vi "Main.vi"() -> ()   [LabVIEW 2017]
uses:
  Controls/Timing Controls.ctl
  Controls/File Controls.ctl
  Controls/DAQ State.ctl
  <vilib>/DAQmx/write.llb/DAQmx Write (Analog 1D DBL NChan 1Samp).vi
  <vilib>/DAQmx/configure/timing.llb/DAQmx Timing (Sample Clock).vi
  <vilib>/DAQmx/miscellaneous.llb/DAQmx Fill In Error Info.vi
panel:
  in  "Single Channel?":bool
  in  "Lower Limit":dbl=-0.85
  in  "Upper Limit":dbl=-0.75
  out "Differential":cluster{dbl[], dbl[]}[](graph)=[{[0.0, 1.0], [0.0029010882279960626, 0.00862868344710327]}, {[-1.0, 2.0], [-0.75, -0.75]}, {[-1.0, 2.0], [-0.85, -0.85]}]
  out "Saving?":bool
  out "Zero Values Dev2":dbl[](array[numeric])
  out "Zero Values Dev1":dbl[](array[numeric])
  in  "Save":bool
  in  "File Control":T1={"File Path"=path "C:/Users/localadmin/Documents/Acquisition Data", "File Name"=""}
  out "Trigger":dynamicdata(graph)=[{"t0"=timestamp(3616576961.7901273 s since 1904-01-01), "dt"=0.001, "Y"=[2.8935987566836108, 2.892940411376444, 2.8932695840305964, 2.8932695840305964, 2.8932695840305964, 2.8932695840305964, 2.8934341703572457, 2.8935987566836108, 2.8935987566836108, 2.893763343009691, 2.8934341703572457, 2.8940925156609985, 2.8940925156609985, 2.8942571019862253, 2.8940925156609985, 2.8935987566836108, 2.893927929335487, 2.893763343009691, 2.893763343009691, 2.8934341703572457, 2.8932695840305964, 2.8932695840305964, 2.8931049977036625, 2.8934341703572457, 2.8931049977036625, 2.8932695840305964, 2.8931049977036625, 2.8935987566836108, 2.893927929335487, 2.893927929335487, 2.893763343009691, 2.8942571019862253, 2.8942571019862253, 2.8940925156609985, 2.893927929335487, 2.893927929335487, 2.893763343009691, 2.893763343009691, 2.8935987566836108, 2.8932695840305964, 2.8934341703572457, 2.892775825048941, 2.8931049977036625, 2.892940411376444, 2.8931049977036625, 2.8934341703572457, 2.8934341703572457, 2.893763343009691, 2.893763343009691, 2.893927929335487, 2.893763343009691, 2.894421688311168, 2.8942571019862253, 2.894421688311168, 2.8940925156609985, 2.893927929335487, 2.894421688311168, 2.894421688311168, 2.893763343009691, 2.8934341703572457, 2.893927929335487, 2.892940411376444, 2.8935987566836108, 2.8931049977036625, 2.8934341703572457, 2.8935987566836108, 2.8935987566836108, 2.893763343009691, 2.893763343009691, 2.8942571019862253, 2.893927929335487, 2.894421688311168, 2.8947508609601993, 2.894421688311168, 2.8940925156609985, 2.8940925156609985, 2.8942571019862253, 2.8940925156609985, 2.893763343009691, 2.8935987566836108, 2.8934341703572457, 2.8931049977036625, 2.892940411376444, 2.8931049977036625, 2.8932695840305964, 2.8931049977036625, 2.8932695840305964, 2.8935987566836108, 2.8935987566836108, 2.8942571019862253, 2.893927929335487, 2.894421688311168, 2.893927929335487, 2.894586274635826, 2.893927929335487, 2.8942571019862253, 2.893927929335487, 2.8940925156609985, 2.893763343009691, 2.8932695840305964], "attributes"=variant("NI_ChannelName"=variant(string "Trigger"), "NI_UnitDescription"=variant(string "Volts"))}]
  out "Dev1":dynamicdata(graph)=[{"t0"=timestamp(3616576961.790079 s since 1904-01-01), "dt"=0.001, "Y"=[0.004713341620051992, 0.0045485913126213084, 0.005042842234350253, 0.0052075925412182755, 0.004219090697197281, 0.0038895900810222983, 0.004219090697197281, 0.0043838410050032195, 0.0038895900810222983, 0.0037248397726536986, 0.004713341620051992, 0.0045485913126213084, 0.0045485913126213084, 0.004054340389203492, 0.0038895900810222983, 0.004713341620051992, 0.004713341620051992, 0.003395339155353394, 0.004878091927295269, 0.004219090697197281, 0.0038895900810222983, 0.003395339155353394, 0.004219090697197281, 0.004713341620051992, 0.0030658385373025787, 0.003395339155353394, 0.0038895900810222983, 0.003395339155353394, 0.0038895900810222983, 0.003230588846421689, 0.003560089464097249, 0.003230588846421689, 0.002571587608819481, 0.003230588846421689, 0.0029010882279960626, 0.0037248397726536986, 0.0030658385373025787, 0.0037248397726536986, 0.0037248397726536986, 0.003560089464097249, 0.003230588846421689, 0.0037248397726536986, 0.003230588846421689, 0.0027363379185016967, 0.0027363379185016967, 0.002571587608819481, 0.003230588846421689, 0.003560089464097249, 0.0037248397726536986, 0.0029010882279960626, 0.0037248397726536986, 0.003395339155353394, 0.003560089464097249, 0.003395339155353394, 0.0038895900810222983, 0.0029010882279960626, 0.003230588846421689, 0.0030658385373025787, 0.0027363379185016967, 0.003395339155353394, 0.0030658385373025787, 0.004054340389203492, 0.003560089464097249, 0.0037248397726536986, 0.0029010882279960626, 0.003230588846421689, 0.002571587608819481, 0.0027363379185016967, 0.0030658385373025787, 0.004054340389203492, 0.0027363379185016967, 0.00240683729894986, 0.002571587608819481, 0.0019125863682161182, 0.0027363379185016967, 0.0029010882279960626, 0.0030658385373025787, 0.0027363379185016967, 0.0030658385373025787, 0.0029010882279960626, 0.00240683729894986, 0.0030658385373025787, 0.0027363379185016967, 0.00240683729894986, 0.002571587608819481, 0.0030658385373025787, 0.003230588846421689, 0.002571587608819481, 0.002242086988892833, 0.003230588846421689, 0.002242086988892833, 0.002242086988892833, 0.0030658385373025787, 0.002571587608819481, 0.003230588846421689, 0.002571587608819481, 0.00240683729894986, 0.004054340389203492, 0.0029010882279960626, 0.0029010882279960626], "attributes"=variant("NI_ChannelName"=variant(string "Dev1_Ch3"), "NI_UnitDescription"=variant(string "Volts"))}] caption="Left"
  out "Dev2":dynamicdata(graph)=[{"t0"=timestamp(3616576961.790079 s since 1904-01-01), "dt"=0.001, "Y"=[0.009451638432940113, 0.009780820425324716, 0.009122456439441123, 0.009122456439441123, 0.010439184406750929, 0.009451638432940113, 0.009451638432940113, 0.009616229429271705, 0.00928704743632991, 0.00862868344710327, 0.008793274444827803, 0.008957865442273755, 0.009122456439441123, 0.009122456439441123, 0.009451638432940113, 0.009451638432940113, 0.00862868344710327, 0.00928704743632991, 0.008464092449100152, 0.009451638432940113, 0.008464092449100152, 0.008957865442273755, 0.01027459341181225, 0.009780820425324716, 0.009780820425324716, 0.00928704743632991, 0.009780820425324716, 0.00862868344710327, 0.00928704743632991, 0.009780820425324716, 0.008957865442273755, 0.00862868344710327, 0.009122456439441123, 0.00928704743632991, 0.00928704743632991, 0.00994541142109917, 0.008299501450818425, 0.00928704743632991, 0.009122456439441123, 0.009451638432940113, 0.009780820425324716, 0.009122456439441123, 0.008957865442273755, 0.009451638432940113, 0.008793274444827803, 0.009780820425324716, 0.009451638432940113, 0.009451638432940113, 0.00928704743632991, 0.008793274444827803, 0.00928704743632991, 0.008957865442273755, 0.007805728454301802, 0.009122456439441123, 0.009451638432940113, 0.00862868344710327, 0.009780820425324716, 0.010110002416595015, 0.008957865442273755, 0.009616229429271705, 0.009122456439441123, 0.009122456439441123, 0.008957865442273755, 0.008957865442273755, 0.00928704743632991, 0.008299501450818425, 0.009122456439441123, 0.009451638432940113, 0.00797031945341925, 0.009451638432940113, 0.009780820425324716, 0.009451638432940113, 0.00928704743632991, 0.009616229429271705, 0.009616229429271705, 0.009616229429271705, 0.009616229429271705, 0.00928704743632991, 0.008793274444827803, 0.008957865442273755, 0.009780820425324716, 0.009122456439441123, 0.008957865442273755, 0.009780820425324716, 0.008134910452258143, 0.009122456439441123, 0.009451638432940113, 0.00928704743632991, 0.00862868344710327, 0.009616229429271705, 0.008134910452258143, 0.009122456439441123, 0.009122456439441123, 0.00928704743632991, 0.008957865442273755, 0.00862868344710327, 0.009122456439441123, 0.008793274444827803, 0.009451638432940113, 0.00862868344710327], "attributes"=variant("NI_ChannelName"=variant(string "Dev2_Ch3"), "NI_UnitDescription"=variant(string "Volts"))}] caption="Right"
  in  "Zero Dev2":bool caption="Zero"
  in  "Zero Dev1":bool caption="Zero"
  in  "Timing":T2={"Sampling Rate (Hz)"=1000.0, "Display Rate (Hz)"=100.0, "Sampling Mode"=10123} {"Sampling Mode" items=["Finite Samples"=10178, "Continuous Samples"=10123, "Hardware Timed Single Point"=12522]; "Sampling Rate (Hz)" format="%0.2f"}
  in  "Run":bool
  out "DAQ \nConnected?":bool
  in  "stop":bool
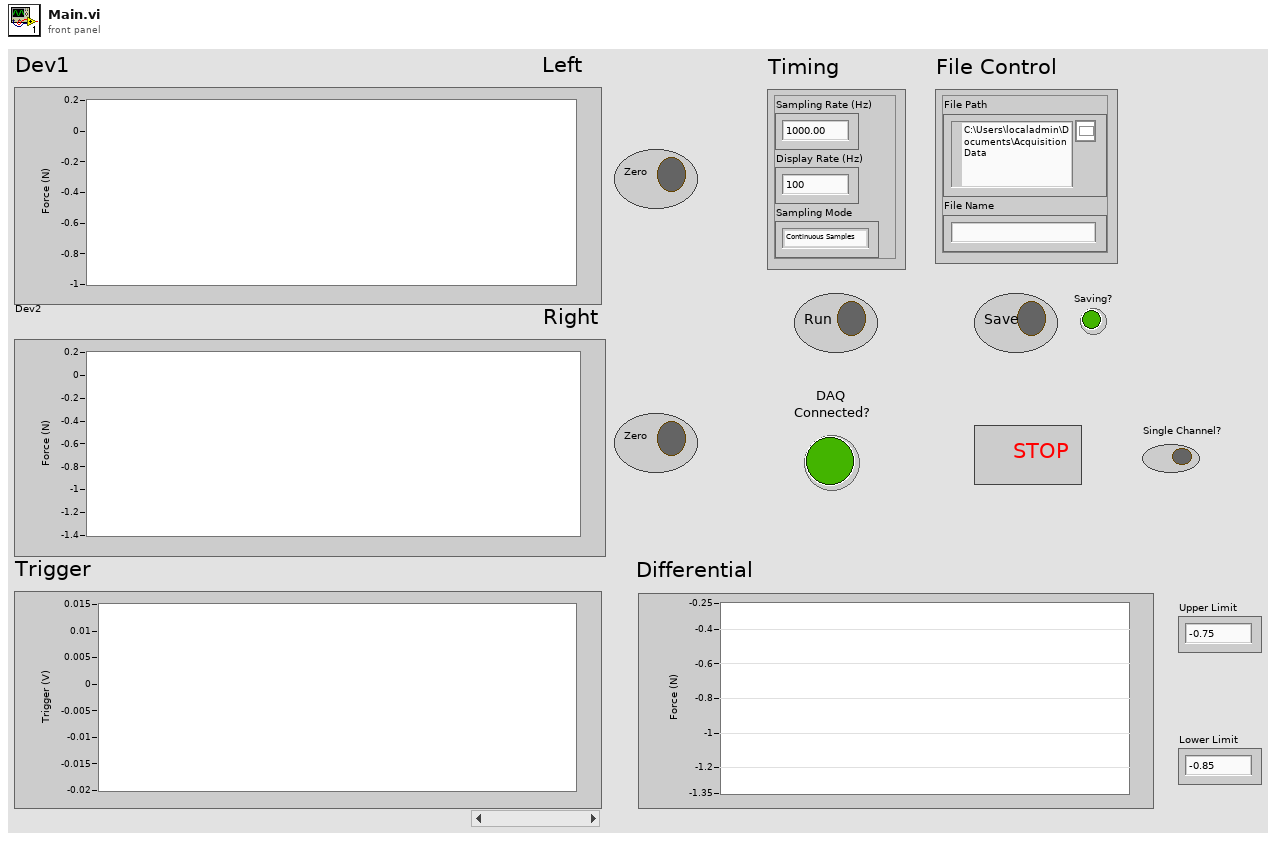
[diagram p1: front panel]
types:
  T1 = typedef "File Controls.ctl" = cluster{"File Path":path, "File Name":string}
  T2 = typedef "Timing Controls.ctl" = cluster{"Sampling Rate (Hz)":dbl, "Display Rate (Hz)":dbl, "Sampling Mode":i32}
  T3 = cluster{"Waveform Array":waveform(dbl)[][], bool}
  T4 = typedef "DAQ State.ctl" = enum16{"Init", "Wait", "Update Timing", "Zero Dev1", "Zero Dev2", "Start Task", "Read", "Stop Task", "Display Data", "Write to File", "Error Handling", "Shutdown"}
  T5 = enum8{"Enabled", "Disabled", "Disabled and Grayed Out"}
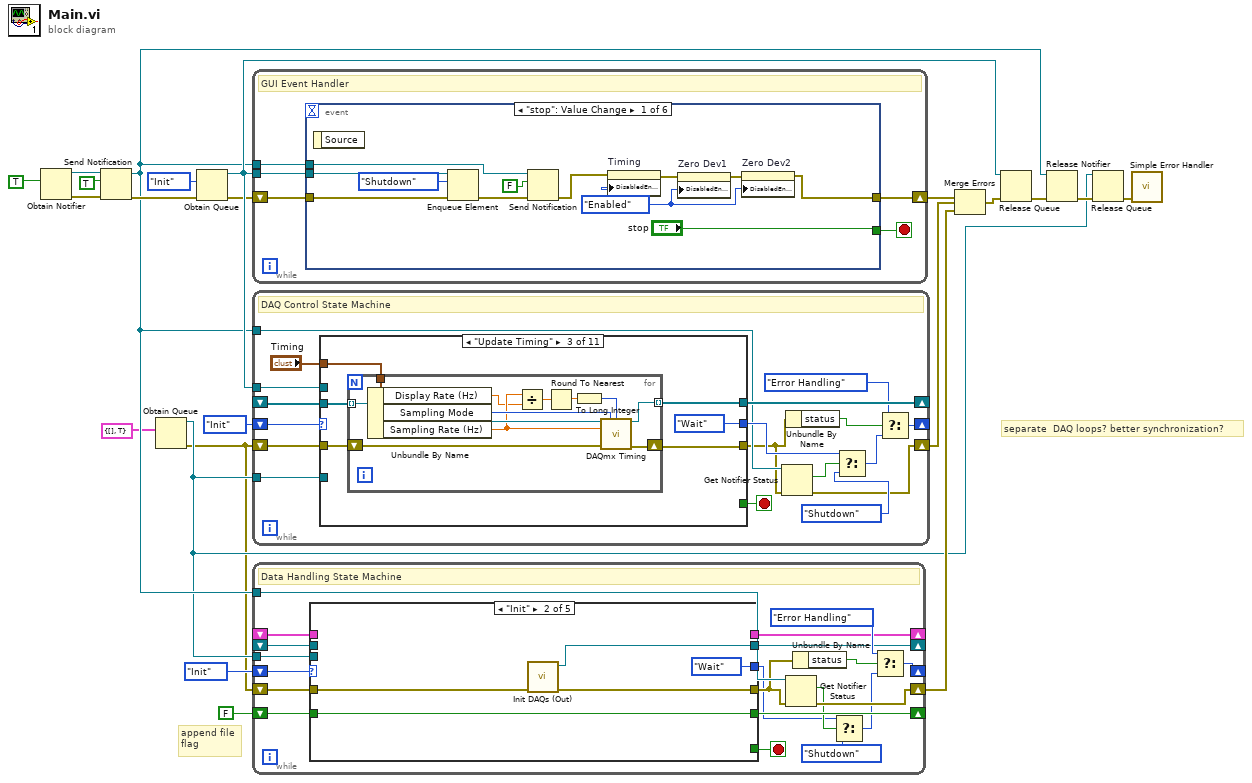
[diagram p0: block diagram]
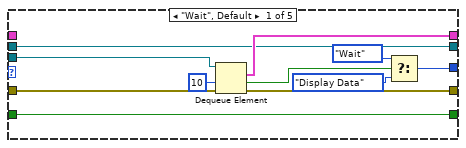
[diagram p2: hidden frame]
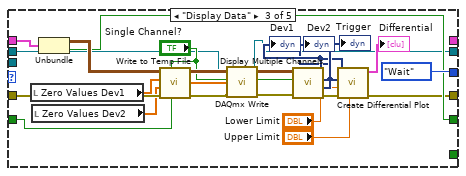
[diagram p3: hidden frame]
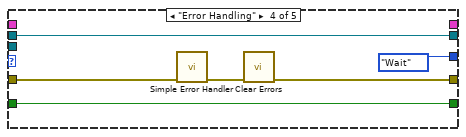
[diagram p4: hidden frame]
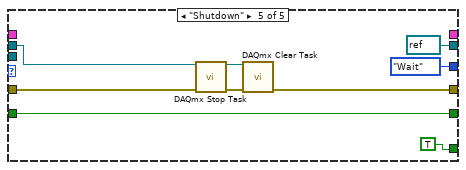
[diagram p5: hidden frame]
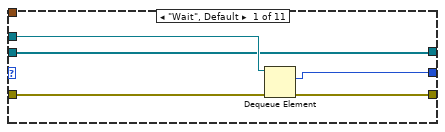
[diagram p6: hidden frame]
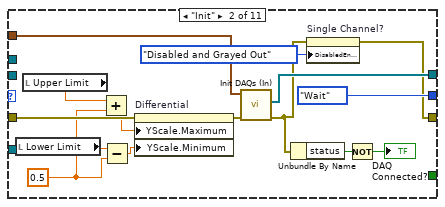
[diagram p7: hidden frame]
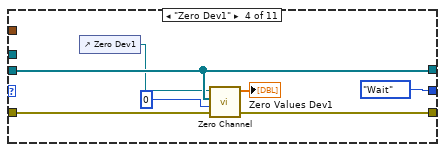
[diagram p8: hidden frame]
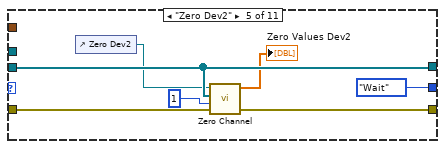
[diagram p9: hidden frame]
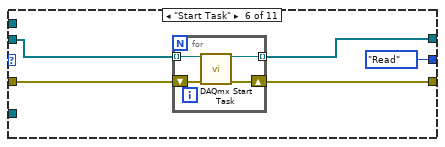
[diagram p10: hidden frame]
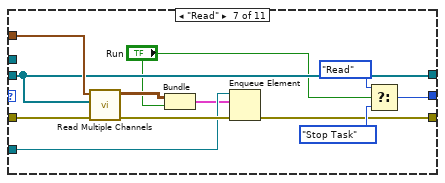
[diagram p11: hidden frame]
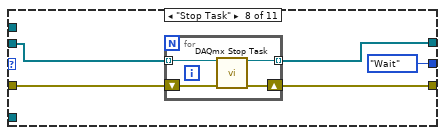
[diagram p12: hidden frame]
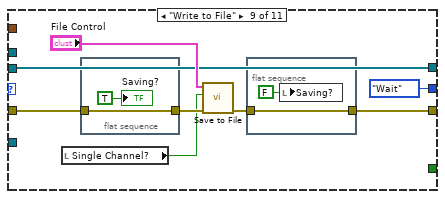
[diagram p13: hidden frame]
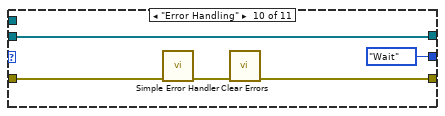
[diagram p14: hidden frame]
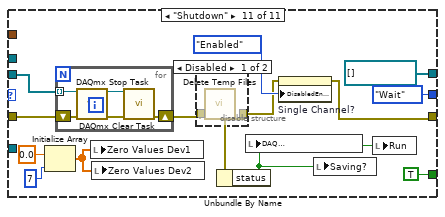
[diagram p15: hidden frame]
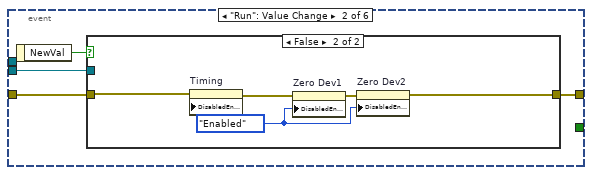
[diagram p17: hidden frame]
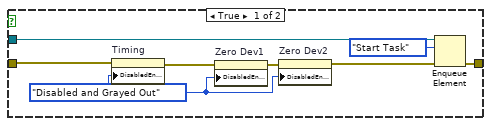
[diagram p18: hidden frame]
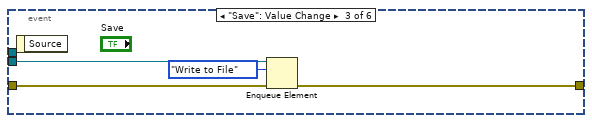
[diagram p19: hidden frame]
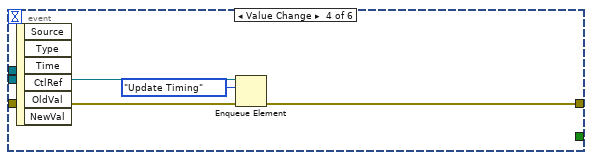
[diagram p20: hidden frame]
diagram:
  # "append file\nflag"
  # "separate  DAQ loops? better synchronization?"
  n1 = Obtain Notifier(notification data type=TRUE) -> (notifier out=w13:refnum<notifier>, error out=w12:errorcluster)  [unwired: 3 in, 1 out]
  n2 = Send Notification(notification=TRUE, notifier=w13, error in (no error)=w12) -> (notifier out=w9:refnum<notifier>, error out=w11:errorcluster)
  n3 = Obtain Queue(element data type=T3 {"Waveform Array"=[], TRUE}) -> (queue out=w6:refnum<queue>, error out=w2:errorcluster)  [unwired: 4 in, 1 out]
  n4 = Obtain Queue(element data type=DAQ_State."Init" ("DAQ State"), error in (no error)=w11) -> (queue out=w17:refnum<queue>, error out=w16:errorcluster)  [unwired: 3 in, 1 out]
  n5 = while {
    tunnel: w17 -> [w26]
    shift-right: [w24] -> w19
    shift-left: w16 -> [w25]
    tunnel: w9 -> [w23]
    stop <- w27 stop-if-true
    # "GUI Event Handler"
    n6 = event shown="[0] \"stop\": Value Change" {
      selector: _ -> [_ _ _ _ _ _]
      dyn-events: _ -> [_ _ _ _ _ _]
      timeout: _ -> [_ _ _ _ _ _]
      tunnel: ["stop" _ _ _ _ _] -> w27
      tunnel: w26 -> [w37 w41 w58 w62 w66 w75]
      tunnel: w25 -> [w38 w43 w60 w63 w67 w76]
      tunnel: [w28 w42 w59 w64 w68 w77] -> w24
      tunnel: w23 -> [w34 _ _ _ _ _]
      event "stop": Value Change {
        w30 = T5."Enabled" ("Disabled")
        n7 = event-data() -> ()  [unwired: 1 in, 1 out]
        n8 = Enqueue Element(queue=w37, element=DAQ_State."Shutdown", error in (no error)=w38) -> (error out=w35:errorcluster)  [unwired: 1 in, 2 out]
        n9 = Send Notification(notification=FALSE, notifier=w34, error in (no error)=w35) -> (error out=w29:errorcluster)  [unwired: 1 out]
        n10 = property on="Timing" class="Clust (strict)"(error in=w29, "DisabledEnum"=w30) -> (error out=w31:errorcluster)  [unwired: 1 in, 1 out]
        n11 = property on="Zero Dev1" class="Bool (strict)"(error in=w31, "DisabledEnum"=w30) -> (error out=w32:errorcluster)  [unwired: 1 in, 1 out]
        n12 = property on="Zero Dev2" class="Bool (strict)"(error in=w32, "DisabledEnum"=w30) -> (error out=w28:errorcluster)  [unwired: 1 in, 1 out]
      }
      event "Run": Value Change {
        n13 = event-data() -> ("NewVal"=w40:bool)  [unwired: 1 in]
        n14 = case shown="False" w40 {
          tunnel: w43 -> [w48 w56]
          tunnel: [w51 w52] -> w42
          tunnel: w41 -> [w50 _]
          frame True {
            w44 = T5."Disabled and Grayed Out" ("Disabled")
            n15 = property on="Timing" class="Clust (strict)"(error in=w48, "DisabledEnum"=w44) -> (error out=w46:errorcluster)  [unwired: 1 in, 1 out]
            n16 = property on="Zero Dev1" class="Bool (strict)"(error in=w46, "DisabledEnum"=w44) -> (error out=w47:errorcluster)  [unwired: 1 in, 1 out]
            n17 = property on="Zero Dev2" class="Bool (strict)"(error in=w47, "DisabledEnum"=w44) -> (error out=w45:errorcluster)  [unwired: 1 in, 1 out]
            n18 = Enqueue Element(queue=w50, element=DAQ_State."Start Task", error in (no error)=w45) -> (error out=w51:errorcluster)  [unwired: 1 in, 2 out]
          }
          frame False {
            w53 = T5."Enabled" ("Disabled")
            n19 = property on="Timing" class="Clust (strict)"(error in=w56, "DisabledEnum"=w53) -> (error out=w54:errorcluster)  [unwired: 1 in, 1 out]
            n20 = property on="Zero Dev1" class="Bool (strict)"(error in=w54, "DisabledEnum"=w53) -> (error out=w55:errorcluster)  [unwired: 1 in, 1 out]
            n21 = property on="Zero Dev2" class="Bool (strict)"(error in=w55, "DisabledEnum"=w53) -> (error out=w52:errorcluster)  [unwired: 1 in, 1 out]
          }
        }
      }
      event "Save": Value Change {
        n22 = event-data() -> ()  [unwired: 1 in, 1 out]
        n23 = Enqueue Element(queue=w58, element=DAQ_State."Write to File", error in (no error)=w60) -> (error out=w59:errorcluster)  [unwired: 1 in, 2 out]
      }
      event Value Change {
        n24 = event-data() -> ()  [unwired: 1 in, 6 out]
        n25 = Enqueue Element(queue=w62, element=DAQ_State."Update Timing", error in (no error)=w63) -> (error out=w64:errorcluster)  [unwired: 1 in, 2 out]
      }
      event "Zero Dev2": Value Change {
        n26 = event-data() -> ()  [unwired: 1 in, 1 out]
        n27 = case shown="False" "Zero Dev2" {
          tunnel: [w69 w72] -> w68
          tunnel: w67 -> [w69 w71]
          tunnel: w66 -> [_ w70]
          frame False {
          }
          frame True {
            n28 = Enqueue Element(queue=w70, element=DAQ_State."Zero Dev2", error in (no error)=w71) -> (error out=w72:errorcluster)  [unwired: 1 in, 2 out]
          }
        }
      }
      event "Zero Dev1": Value Change {
        n29 = event-data() -> ()  [unwired: 1 in, 1 out]
        n30 = case shown="True" "Zero Dev1" {
          tunnel: [w78 w81] -> w77
          tunnel: w76 -> [w78 w80]
          tunnel: w75 -> [_ w79]
          frame False {
          }
          frame True {
            n31 = Enqueue Element(queue=w79, element=DAQ_State."Zero Dev1", error in (no error)=w80) -> (error out=w81:errorcluster)  [unwired: 1 in, 2 out]
          }
        }
      }
    }
  }
  n32 = while {
    shift-right: [w93] -> _
    shift-left: DAQ_State."Init" ("DAQ State") -> [w100]
    shift-right: [w84] -> w20
    shift-left: w2 -> [w99]
    tunnel: w17 -> [w97]
    shift-right: [w96] -> _
    shift-left: _ -> [w95]
    tunnel: w6 -> [w87]
    tunnel: w9 -> [w86]
    stop <- w98 stop-if-true
    # "DAQ Control State Machine"
    n33 = case shown="\"Update Timing\"" w100 {
      tunnel: [w102 DAQ_State."Wait" ("DAQ State") DAQ_State."Wait" ("DAQ State") DAQ_State."Wait" ("DAQ State") DAQ_State."Wait" ("DAQ State") DAQ_State."Read" ("DAQ State") w170 DAQ_State."Wait" ("DAQ State") DAQ_State."Wait" ("DAQ State") DAQ_State."Wait" ("DAQ State") DAQ_State."Wait" ("DAQ State")] -> w90
      tunnel: [w105 w106 w125 w143 w150 w155 w164 w176 w185 w197 w200] -> w85
      tunnel: w99 -> [w104 w115 w126 w144 w151 w156 w172 w173 w184 w198 w210]
      tunnel: [_ _ _ _ _ _ _ _ _ _ TRUE] -> w98
      tunnel: w97 -> [w103 _ _ _ _ _ _ _ _ _ _]
      tunnel: [w101 w116 w121 w142 w149 w153 w167 w177 w187 w194 refnum<k21>[] [] ("Channel Array")] -> w96
      tunnel: w95 -> [w101 _ w122 w142 w149 w154 w167 w174 w187 w194 w208]
      tunnel: "Timing" -> [_ w117 w123 _ _ _ w168 _ _ _ _]
      tunnel: w87 -> [_ _ _ _ _ _ w165 _ _ _ _]
      frame "Wait", Default {
        n34 = Dequeue Element(queue=w103, error in (no error)=w104) -> (element=w102:T4, error out=w105:errorcluster)  [unwired: 1 in, 2 out]
      }
      frame "Init" {
        w110 = 0.5 ("Y Scale.Range:Maximum")
        n35 = local read "Lower Limit"() -> (w113:dbl)
        n36 = local read "Upper Limit"() -> (w111:dbl)
        n37 = Add(x=w111, y=w110) -> (x+y=w109:dbl)
        n38 = Subtract(x=w113, y=w110) -> (x-y=w112:dbl)
        n39 = property on="Differential" class="XYGraph (strict)"(error in=w115, "YScale.Maximum"=w109, "YScale.Minimum"=w112) -> (error out=w114:errorcluster)  [unwired: 1 in, 1 out]
        n40 = call "Init DAQs (In).vi"("error in (no error)"=w114, "Timing"=w117) -> ("error out"=w107:errorcluster, "Channel Array"=w116:refnum<k21>[])  [unwired: 8 in]
        n41 = Unbundle By Name(w107) -> ("status"=w119:bool)
        n42 = property on="Single Channel?" class="Bool (strict)"(error in=w107, "DisabledEnum"=T5."Disabled and Grayed Out" ("Disabled")) -> (error out=w106:errorcluster)  [unwired: 1 in, 1 out]
        n43 = Not(x=w119) -> (.not. x?=→"DAQ \nConnected?":bool)
      }
      frame "Update Timing" {
        n44 = for {
          shift-right: [w136] -> w125
          shift-left: w126 -> [w137]
          tunnel: [w135] -> w121 mode=indexing
          tunnel: w123 -> [w134]
          tunnel: w122 -> [w132] mode=indexing
          n45 = Unbundle By Name(w134) -> ("Display Rate (Hz)"=w130:dbl, "Sampling Mode"=w133:i32, "Sampling Rate (Hz)"=w131:dbl)
          n46 = Divide(x=w131, y=w130) -> (x/y=w129:dbl)
          n47 = Round To Nearest(number=w129) -> (nearest integer value=w128:dbl)
          n48 = To Long Integer(number=w128) -> (32bit integer=w127:i32)
          n49 = call-poly <vilib>:"DAQmx Timing.vi"("task/channels in"=w132, "sample mode"=w133, "samples per channel"=w127, "rate"=w131, "error in"=w137) -> ("task out"=w135:refnum<k21>, "error out"=w136:errorcluster)  [unwired: 9 in]
        }
      }
      frame "Zero Dev1" {
        n50 = control-ref of="Zero Dev1"() -> (w140:refnum<vi>)
        n51 = call "Zero Channel.vi"("error in (no error)"=w144, "Dev to Zero"=0, "Channel Array"=w142, "Refnum"=w140) -> ("error out"=w143:errorcluster, "Zero Values"=→"Zero Values Dev1":dbl[])  [unwired: 6 in]
      }
      frame "Zero Dev2" {
        n52 = control-ref of="Zero Dev2"() -> (w147:refnum<vi>)
        n53 = call "Zero Channel.vi"("error in (no error)"=w151, "Dev to Zero"=1, "Channel Array"=w149, "Refnum"=w147) -> ("error out"=w150:errorcluster, "Zero Values"=→"Zero Values Dev2":dbl[])  [unwired: 6 in]
      }
      frame "Start Task" {
        n54 = for {
          shift-right: [w159] -> w155
          shift-left: w156 -> [w160]
          tunnel: w154 -> [w158] mode=indexing
          tunnel: [w157] -> w153 mode=indexing
          n55 = call <vilib>:"DAQmx Start Task.vi"("task/channels in"=w158, "error in"=w160) -> ("task out"=w157:refnum<k21>, "error out"=w159:errorcluster)  [unwired: 12 in]
        }
      }
      frame "Read" {
        n56 = call "Read Multiple Channels.vi"("error in (no error)"=w172, "Channel Array"=w167, "Timing"=w168) -> ("error out"=w166:errorcluster, "data"=w162:waveform(dbl)[][])  [unwired: 7 in]
        n57 = Bundle("data"=w162, "Run"="Run") -> (w163:cluster{"data":waveform(dbl)[][], "Run":bool})  [unwired: 1 in]
        n58 = Enqueue Element(queue=w165, element=w163, error in (no error)=w166) -> (error out=w164:errorcluster)  [unwired: 1 in, 2 out]
        n59 = Select(t=DAQ_State."Read", s="Run", f=DAQ_State."Stop Task" ("DAQ State")) -> (s? t:f=w170:T4)
      }
      frame "Stop Task" {
        n60 = for {
          shift-right: [w179] -> w176
          shift-left: w173 -> [w180]
          tunnel: w174 -> [w181] mode=indexing
          tunnel: [w178] -> w177 mode=indexing
          n61 = call <vilib>:"DAQmx Stop Task.vi"("task/channels in"=w181, "error in"=w180) -> ("task out"=w178:refnum<k21>, "error out"=w179:errorcluster)  [unwired: 12 in]
        }
      }
      frame "Write to File" {
        n62 = local read "Single Channel?"() -> (w182:bool)
        n63 = flat-sequence {
          tunnel: w184 -> [w191]
          tunnel: [w191] -> w183
          frame #0 {
            "Saving?" <- TRUE ("Saving?")
          }
        }
        n64 = call "Save to File.vi"("error in (no error)"=w183, "Single Channel?"=w182, "File Control"="File Control") -> ("error out"=w186:errorcluster)  [unwired: 8 in]
        n65 = flat-sequence {
          tunnel: w186 -> [w193]
          tunnel: [w193] -> w185
          frame #0 {
            n66 = local write "Saving?"(FALSE ("Saving?")) -> ()
          }
        }
      }
      frame "Error Handling" {
        n67 = call <vilib>:"Simple Error Handler.vi"("error in (no error)"=w198) -> ("error out"=w196:errorcluster)  [unwired: 4 in, 4 out]
        n68 = call <vilib>:"Clear Errors.vi"("error in (no error)"=w196) -> ("error out"=w197:errorcluster)  [unwired: 5 in, 1 out]
      }
      frame "Shutdown" {
        n69 = Initialize Array(0.0 ("element"), 7 ("dimension size")) -> (w205:dbl[])
        n70 = for {
          shift-right: [w219] -> w206
          shift-left: w210 -> [w216]
          tunnel: w208 -> [w218] mode=indexing
          n71 = call <vilib>:"DAQmx Stop Task.vi"("task/channels in"=w218, "error in"=w216) -> ("task out"=w217:refnum<k21>, "error out"=w215:errorcluster)  [unwired: 12 in]
          n72 = call <vilib>:"DAQmx Clear Task.vi"("task in"=w217, "error in"=w215) -> ("error out"=w219:errorcluster)  [unwired: 13 in]
        }
        n73 = local write "Zero Values Dev1"(w205) -> ()
        n74 = local write "Zero Values Dev2"(w205) -> ()
        n75 = disable-structure shown="Disabled" {
          disable-tunnel: w206 -> [w213 w214]
          disable-tunnel: [w212 w214] -> w199
          frame Disabled {
            n76 = call "Delete Temp Files.vi"("error in (no error)"=w213) -> ("error out"=w212:errorcluster)  [unwired: 10 in]
          }
          frame Enabled {
          }
        }
        n77 = Unbundle By Name(w206) -> ("status"=w202:bool)
        n78 = local write "DAQ \nConnected?"(w202) -> ()
        n79 = property on="Single Channel?" class="Bool (strict)"(error in=w199, "DisabledEnum"=T5."Enabled" ("Disabled")) -> (error out=w200:errorcluster)  [unwired: 1 in, 1 out]
        n80 = local write "Saving?"(w202) -> ()
        n81 = local write "Run"(w202) -> ()
      }
    }
    n82 = Get Notifier Status(notifier=w86, error in (no error)=w85) -> (current notification=w83:bool, error out=w84:errorcluster)  [unwired: 3 out]
    n83 = Unbundle By Name(w85) -> ("status"=w94:bool)
    n84 = Select(t=w90, s=w83, f=DAQ_State."Shutdown" ("t")) -> (s? t:f=w89:T4)
    n85 = Select(t=DAQ_State."Error Handling", s=w94, f=w89) -> (s? t:f=w93:T4)
  }
  n86 = while {
    shift-right: [w229] -> _
    shift-left: DAQ_State."Init" ("DAQ State") -> [w239]
    shift-right: [w232] -> w7
    shift-left: w2 -> [w238]
    tunnel: w9 -> [w237]
    tunnel: w6 -> [w236]
    shift-right: [w231] -> _
    shift-left: _ -> [w230]
    shift-right: [w227] -> _
    shift-left: FALSE ("Append to file?") -> [w228]
    shift-right: [w226] -> _
    shift-left: _ -> [w225]
    stop <- w224 stop-if-true
    # "Data Handling State Machine"
    n87 = case shown="\"Init\"" w239 {
      tunnel: w238 -> [w250 w255 w276 w283 w292]
      tunnel: [w249 w254 w262 w282 w290] -> w233
      tunnel: w236 -> [w248 _ _ _ _]
      tunnel: [w243 DAQ_State."Wait" ("t") DAQ_State."Wait" ("t") DAQ_State."Wait" ("t") DAQ_State."Wait" ("t")] -> w221
      tunnel: [w247 _ _ _ _] -> w231
      tunnel: w230 -> [_ _ w275 _ _]
      tunnel: w228 -> [w242 w251 w270 w280 w286]
      tunnel: [w242 w251 w273 w280 w286] -> w227
      tunnel: [w241 w252 w257 w279 refnum<k21> refnum ("task out")] -> w226
      tunnel: w225 -> [w241 _ w258 w279 w289]
      tunnel: [_ _ _ _ TRUE] -> w224
      frame "Wait", Default {
        n88 = Dequeue Element(queue=w248, timeout in ms (-1)=10, error in (no error)=w250) -> (element=w247:T3, timed out?=w246:bool, error out=w249:errorcluster)  [unwired: 1 out]
        n89 = Select(t=DAQ_State."Wait", s=w246, f=DAQ_State."Display Data" ("t")) -> (s? t:f=w243:T4)
      }
      frame "Init" {
        n90 = call "Init DAQs (Out).vi"("error in (no error)"=w255) -> ("error out"=w254:errorcluster, "Channel"=w252:refnum<k21>)  [unwired: 9 in]
      }
      frame "Display Data" {
        n91 = local read "Zero Values Dev1"() -> (w272:dbl[])
        n92 = local read "Zero Values Dev2"() -> (w271:dbl[])
        n93 = Unbundle(w275) -> ("Waveform Array"=w274:waveform(dbl)[][], w273:bool)
        n94 = call "Write to Temp File.vi"("Append to file?"=w270, "Single Channel?"="Single Channel?", "error in (no error)"=w276, "Dev2 Zero Values"=w271, "Dev1 Zero Values"=w272, "Waveform Array"=w274) -> ("error out"=w260:errorcluster, "Force Outputs"=w256:dbl[], "Zeroed Array"=w269:waveform(dbl)[][])  [unwired: 3 in]
        n95 = call-poly <vilib>:"DAQmx Write.vi"("task/channels in"=w258, "data"=w256, "error in"=w260) -> ("task out"=w257:refnum<k21>, "error out"=w259:errorcluster)  [unwired: 10 in, 1 out]
        n96 = call "Display Multiple Channels.vi"("Error In"=w259, "Single Channel?"="Single Channel?", "Waveform Array"=w269) -> ("Error Out"=w263:errorcluster, "Trigger"=→"Trigger":dynamicdata, "Dev2 Ch3"=w267:dynamicdata, "Dev1 Ch3"=w268:dynamicdata)  [unwired: 5 in]
        "Dev1" <- w268
        "Dev2" <- w267
        n97 = call "Create Differential Plot.vi"("Upper Limit"="Upper Limit", "Error In"=w263, "Lower Limit"="Lower Limit", "Dev2 Ch3"=w267, "Dev1 Ch3"=w268) -> ("Error Out"=w262:errorcluster, "Array"=→"Differential":cluster{"Array":dbl[], "Array":dbl[]}[])  [unwired: 5 in]
      }
      frame "Error Handling" {
        n98 = call <vilib>:"Simple Error Handler.vi"("error in (no error)"=w283) -> ("error out"=w284:errorcluster)  [unwired: 4 in, 4 out]
        n99 = call <vilib>:"Clear Errors.vi"("error in (no error)"=w284) -> ("error out"=w282:errorcluster)  [unwired: 5 in, 1 out]
      }
      frame "Shutdown" {
        n100 = call <vilib>:"DAQmx Stop Task.vi"("task/channels in"=w289, "error in"=w292) -> ("task out"=w288:refnum<k21>, "error out"=w291:errorcluster)  [unwired: 12 in]
        n101 = call <vilib>:"DAQmx Clear Task.vi"("task in"=w288, "error in"=w291) -> ("error out"=w290:errorcluster)  [unwired: 13 in]
      }
    }
    n102 = Get Notifier Status(notifier=w237, error in (no error)=w233) -> (current notification=w223:bool, error out=w232:errorcluster)  [unwired: 3 out]
    n103 = Unbundle By Name(w233) -> ("status"=w234:bool)
    n104 = Select(t=w221, s=w223, f=DAQ_State."Shutdown") -> (s? t:f=w222:T4)
    n105 = Select(t=DAQ_State."Error Handling", s=w234, f=w222) -> (s? t:f=w229:T4)
  }
  n106 = Merge Errors(w19, w20, w7) -> (w18:errorcluster)
  n107 = Release Queue(queue=w17, error in (no error)=w18) -> (error out=w1:errorcluster)  [unwired: 1 in, 2 out]
  n108 = Release Notifier(notifier=w9, error in (no error)=w1) -> (error out=w8:errorcluster)  [unwired: 1 in, 2 out]
  n109 = Release Queue(queue=w6, error in (no error)=w8) -> (error out=w5:errorcluster)  [unwired: 1 in, 2 out]
  n110 = call <vilib>:"Simple Error Handler.vi"("error in (no error)"=w5) -> ()  [unwired: 4 in, 5 out]
